vi "Exercise 5.2 Webservice Pi Browser.vi"() -> ()   [LabVIEW 2014]
uses:
  <vilib>/Q-Wave Systems/QwaveSys RPi Training Package (Demo)/Addons/QwaveSys RPi Training Library.lvlib
  <vilib>/Q-Wave Systems/QwaveSys RPi Training Package (Demo)/Addons/WiringPi/WiringPi Pin Mode.ctl
  <vilib>/Q-Wave Systems/QwaveSys RPi Training Package/Solutions/Solutions 5 Webservice/temp.vi
  <vilib>/Q-Wave Systems/QwaveSys RPi Training Package/Solutions/Solutions 5 Webservice/led1.vi
  <vilib>/Q-Wave Systems/QwaveSys RPi Training Package/Solutions/Solutions 5 Webservice/led2.vi
  <vilib>/Q-Wave Systems/QwaveSys RPi Training Package (Demo)/Addons/WiringPi/WiringPi GPIO TypeDef.ctl
panel:
  in  "stop":bool
  out "Active":bool
  in  "LED2":T1=5 items=["Pin1_3.3V"=51, "Pin2_5V"=52, "Pin3_GPIO8_I2C1_SDA"=8, "Pin4_5V"=53, "Pin5_GPIO9_I2C1_SCL"=9, "Pin6_Gnd"=54, "Pin7_GPIO7_GPCLK0"=7, "Pin8_GPIO15_TXD_UART"=15, "Pin9_Gnd"=55, "Pin10_GPIO16_RXD_UART"=16, "Pin11_GPIO0"=0, "Pin12_GPIO1_PCMCLK_PWM0"=1, "Pin13_GPIO2"=2, "Pin14_Gnd"=56, "Pin15_GPIO3"=3, "Pin16_GPIO4"=4, "Pin17_3V"=57, "Pin18_GPIO5"=5, "Pin19_GPIO12_MOSI(SPI)"=12, "Pin20_Gnd"=58, "Pin21_GPIO13_MISO(SPI)"=13, "Pin22_GPIO6"=6, "Pin23_GPIO14_CLK(SPI)"=14, "Pin24_GPIO10_CE0_SPI"=10, "Pin25_Gnd"=59, "Pin26_GPIO11_CE1_SPI"=11, "Pin27_SDA0_I2C_EEPROM"=60, "Pin28_SCL0_I2C_EEPROM"=61, "Pin_29_GPIO21_GPCLK1"=21, "Pin30_Gnd"=62, "Pin31_GPIO22_GPCLK2"=22, "Pin32_GPIO26_PWM0"=26, "Pin33_GPIO23_PWM1"=23, "Pin34_Gnd"=63, "Pin35_GPIO24_PCMFS_PWM1"=24, "Pin36_GPIO27"=27, "Pin37_GPIO25"=25, "Pin38_GPIO28_PCM_DIN"=28, "Pin39_Gnd"=64, "Pin40_GPIO29_PCM_DOUT"=29]
  in  "LED1":T1=1 items=["Pin1_3.3V"=51, "Pin2_5V"=52, "Pin3_GPIO8_I2C1_SDA"=8, "Pin4_5V"=53, "Pin5_GPIO9_I2C1_SCL"=9, "Pin6_Gnd"=54, "Pin7_GPIO7_GPCLK0"=7, "Pin8_GPIO15_TXD_UART"=15, "Pin9_Gnd"=55, "Pin10_GPIO16_RXD_UART"=16, "Pin11_GPIO0"=0, "Pin12_GPIO1_PCMCLK_PWM0"=1, "Pin13_GPIO2"=2, "Pin14_Gnd"=56, "Pin15_GPIO3"=3, "Pin16_GPIO4"=4, "Pin17_3V"=57, "Pin18_GPIO5"=5, "Pin19_GPIO12_MOSI(SPI)"=12, "Pin20_Gnd"=58, "Pin21_GPIO13_MISO(SPI)"=13, "Pin22_GPIO6"=6, "Pin23_GPIO14_CLK(SPI)"=14, "Pin24_GPIO10_CE0_SPI"=10, "Pin25_Gnd"=59, "Pin26_GPIO11_CE1_SPI"=11, "Pin27_SDA0_I2C_EEPROM"=60, "Pin28_SCL0_I2C_EEPROM"=61, "Pin_29_GPIO21_GPCLK1"=21, "Pin30_Gnd"=62, "Pin31_GPIO22_GPCLK2"=22, "Pin32_GPIO26_PWM0"=26, "Pin33_GPIO23_PWM1"=23, "Pin34_Gnd"=63, "Pin35_GPIO24_PCMFS_PWM1"=24, "Pin36_GPIO27"=27, "Pin37_GPIO25"=25, "Pin38_GPIO28_PCM_DIN"=28, "Pin39_Gnd"=64, "Pin40_GPIO29_PCM_DOUT"=29]
  out "error out":errorcluster
  in  "error in (no error)":errorcluster
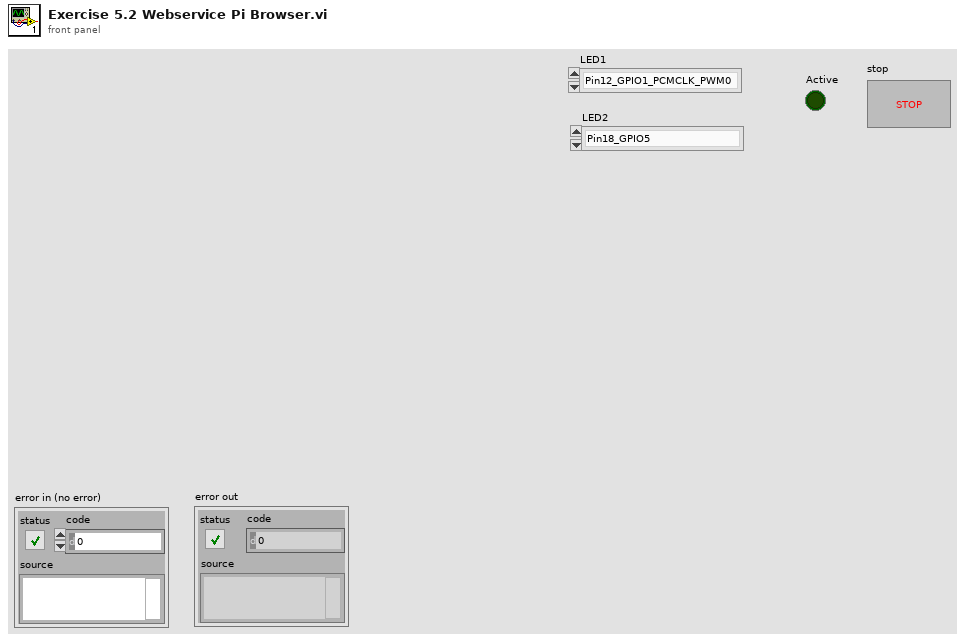
[diagram p1: front panel]
types:
  T1 = typedef "QwaveSys RPi Training Library.lvlib/WiringPi GPIO TypeDef.ctl" = u8
  T2 = typedef "QwaveSys RPi Training Library.lvlib/WiringPi Pin Mode.ctl" = enum8{"INPUT", "OUTPUT", "PWM_OUTPUT", "GPIO_CLOCK", "SOFT_PWM_OUTPUT", "SOFT_TONE_OUTPUT", "PWM_TONE_OUTPUT"}
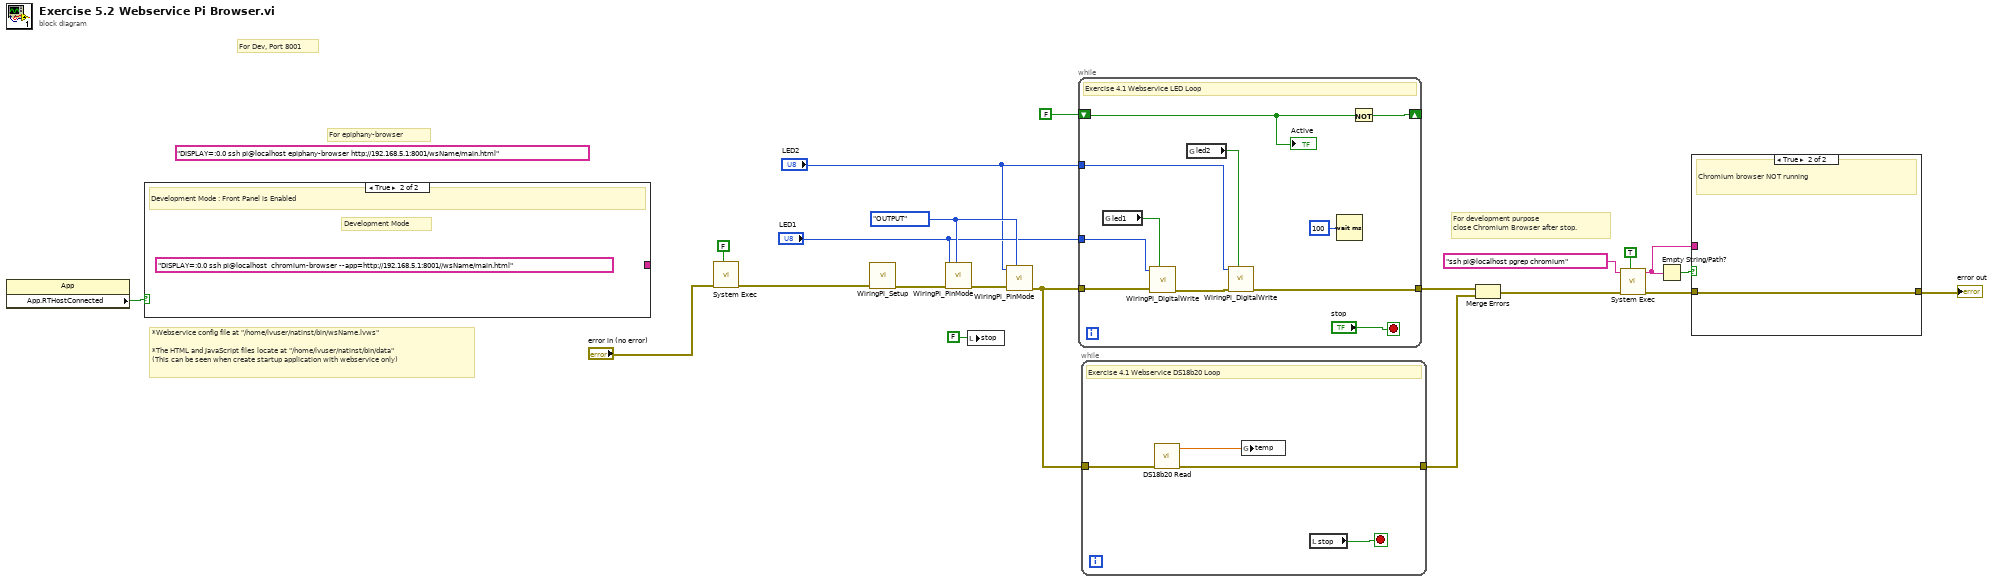
[diagram p0: block diagram]
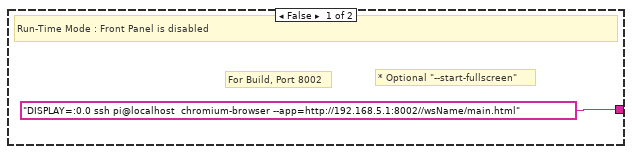
[diagram p2: hidden frame]
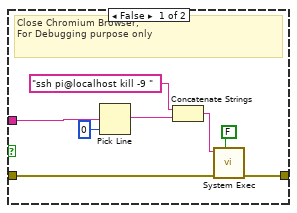
[diagram p3: hidden frame]
diagram:
  (unwired) "DISPLAY=:0.0 ssh pi@localhost epiphany-browser http://192.168.5.1:8001/wsName/main.html" ("command line")
  w19 = WiringPi_Pin_Mode."OUTPUT" ("Pin Mode")
  # "*Webservice config file at \"/home/lvuser/natinst/bin/wsName.lvws\"\n\n*The HTML and JavaScript files locate at \"/home/lvuser/natinst/bin/data\" \n(This can be seen when create startup application with webservice only)"
  # "For development purpose\nclose Chromium Browser after stop."
  # "For epiphany-browser"
  # "For Dev, Port 8001"
  n1 = property class="App"() -> ("App.RTHostConnected"=w1:bool)  [unwired: 2 in, 2 out]
  n2 = case shown="True" w1 {
    tunnel: ["DISPLAY=:0.0 ssh pi@localhost  chromium-browser --app=http://192.168.5.1:8002//wsName/main.html" ("command line") _] -> _
    frame False {
      # "For Build, Port 8002"
      # "* Optional \"--start-fullscreen\""
      # "Run-Time Mode : Front Panel is disabled"
    }
    frame True {
      (unwired) "DISPLAY=:0.0 ssh pi@localhost  chromium-browser --app=http://192.168.5.1:8001//wsName/main.html" ("command line")
      # "Development Mode"
      # "Development Mode : Front Panel is Enabled"
    }
  }
  n3 = call <vilib>:"System Exec.vi"("wait until completion? (T)"=FALSE, "error in (no error)"="error in (no error)") -> ("error out"=w10:errorcluster)  [unwired: 6 in, 3 out]
  n4 = call <vilib>:"WiringPi_Setup.vi"("error in (no error)"=w10) -> ("error out"=w21:errorcluster)  [unwired: 10 in]
  n5 = call <vilib>:"WiringPi_PinMode.vi"("Pin Mode"=w19, "error in (no error)"=w21, "WiringPi GPIO"="LED1") -> ("error out"=w20:errorcluster)  [unwired: 8 in]
  n6 = local write "stop"(FALSE ("stop")) -> ()
  n7 = call <vilib>:"WiringPi_PinMode.vi"("Pin Mode"=w19, "error in (no error)"=w20, "WiringPi GPIO"="LED2") -> ("error out"=w16:errorcluster)  [unwired: 8 in]
  n8 = while {
    tunnel: w16 -> [w32]
    tunnel: "LED1" -> [w31]
    tunnel: "LED2" -> [w30]
    tunnel: [w27] -> w15
    shift-right: [w25] -> _
    shift-left: FALSE -> [w24]
    stop <- "stop" stop-if-true
    # "Exercise 4.1 Webservice LED Loop"
    n9 = global read "led1.vi" "led1"() -> (w29:bool)
    n10 = call <vilib>:"WiringPi_DigitalWrite.vi"("Value"=w29, "error in (no error)"=w32, "WiringPi GPIO"=w31) -> ("error out"=w33:errorcluster)  [unwired: 8 in]
    n11 = global read "led2.vi" "led2"() -> (w28:bool)
    n12 = call <vilib>:"WiringPi_DigitalWrite.vi"("Value"=w28, "error in (no error)"=w33, "WiringPi GPIO"=w30) -> ("error out"=w27:errorcluster)  [unwired: 8 in]
    n13 = Wait (ms)(milliseconds to wait=u32 100) -> ()  [unwired: 1 out]
    n14 = Not(x=w24) -> (.not. x?=w25:bool)
    "Active" <- w24
  }
  n15 = while {
    tunnel: w16 -> [w36]
    tunnel: [w35] -> w14
    stop <- w34 stop-if-true
    # "Exercise 4.1 Webservice DS18b20 Loop"
    n16 = call <vilib>:"DS18b20 Read.vi"("error in (no error)"=w36) -> ("error out"=w35:errorcluster, "Temp"=w37:dbl)  [unwired: 7 in, 2 out]
    n17 = global write "temp.vi" "temp"(w37) -> ()
    n18 = local read "stop"() -> (w34:bool)
  }
  n19 = Merge Errors(w15, w14) -> (w8:errorcluster)
  n20 = call <vilib>:"System Exec.vi"("wait until completion? (T)"=TRUE, "error in (no error)"=w8, "command line"="ssh pi@localhost pgrep chromium") -> ("error out"=w5:errorcluster, "standard output"=w4:string)  [unwired: 5 in, 2 out]
  n21 = Empty String/Path?(string/path=w4) -> (empty?=w6:bool)
  n22 = case shown="True" w6 {
    tunnel: w5 -> [w45 w46]
    tunnel: w4 -> [w44 _]
    tunnel: [w38 w46] -> w3
    frame False {
      # "Close Chromium Browser,\nFor Debugging purpose only"
      n23 = Pick Line(multi-line string=w44, line index=0) -> (output string=w41:string)  [unwired: 1 in]
      n24 = Concatenate Strings("ssh pi@localhost kill -9 " ("command line"), w41) -> (w40:string)
      n25 = call <vilib>:"System Exec.vi"("wait until completion? (T)"=FALSE, "error in (no error)"=w45, "command line"=w40) -> ("error out"=w38:errorcluster)  [unwired: 5 in, 3 out]
    }
    frame True {
      # "Chromium browser NOT running"
    }
  }
  "error out" <- w3
